vi "Global_HW Status.vi"() -> ()   [LabVIEW 2017, in "VisionSystem.lvlib"]
uses:
  VisionSystem.lvlib
  Cluster_HW_Status.ctl
  <vilib>/vision/Image Controls.llb/IMAQ Image.ctl
  TypeDefs/Cluster_Camera Settings.ctl
  <vilib>/Rock Robotics/WPI/Camera/WPI_CameraImageSize.ctl
  <vilib>/Rock Robotics/WPI/Camera/WPI_CameraFrameRate.ctl
  <vilib>/Rock Robotics/WPI/Camera/WPI_CameraWhite Balance Values.ctl
  <vilib>/Rock Robotics/WPI/Camera/WPI_CameraExposure Values.ctl
  Enum_ Field Targets.ctl
  <vilib>/Rock Robotics/WPI/Camera/WPI_CameraDevRef.ctl
panel:
  in  "HW Vision_Status":T1 {"Cam Setings"."Saturation" min=0 max=100 step=1; "Cam Setings"."Sharpness" min=0 max=100 step=1; "Cam Setings"."Brightness" min=0 max=100 step=1; "Cam Setings"."Exposure (%)" min=0.0 max=100.0 step=1.0}
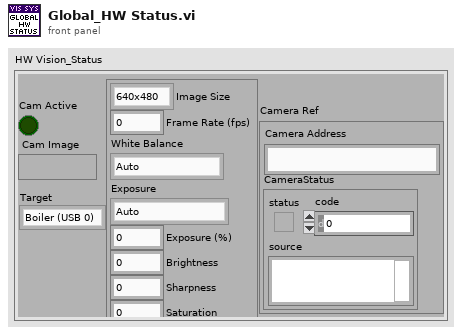
[diagram p1: front panel]
types:
  T1 = typedef "VisionSystem.lvlib/Cluster_HW_Status.ctl" = cluster{"Cam Active":bool, "Cam Image":T2, "Cam Setings":T3, "Target":T8, "Camera Ref":T9}
  T2 = typedef "IMAQ Image.ctl" = refnum<image>
  T3 = typedef "Cluster_Camera Settings.ctl" = cluster{"Image Size":T4, "Frame Rate (fps)":T5, "White Balance":T6, "Exposure":T7, "Exposure (%)":dbl, "Brightness":i32, "Sharpness":i32, "Saturation":i32}
  T4 = typedef "WPI_CameraImageSize.ctl" = enum16{"640x480", "320x240", "160x120", "Custom"}
  T5 = typedef "WPI_CameraFrameRate.ctl" = u32
  T6 = typedef "WPI_CameraWhite Balance Values.ctl" = enum16{"Auto", "Fixed indoor", "Fixed outdoor 1", "Fixed outdoor 2", "Fixed fluorescent 1", "Fixed fluorescent 2", "Hold current", "Custom"}
  T7 = typedef "WPI_CameraExposure Values.ctl" = enum16{"Auto", "Flicker-free 50 Hz", "Flicker-free 60 Hz", "Hold current", "Custom"}
  T8 = typedef "VisionSystem.lvlib/Enum_ Field Targets.ctl" = enum16{"Boiler (USB 0)", "Rope (USB 1)"}
  T9 = typedef "WPI_CameraDevRef.ctl" = cluster{"Camera Address":string, "CameraStatus":errorcluster}
diagram:
